vi "Test_WireLoops.vi"() -> ()   [LabVIEW 2025]
uses:
  8cebb4ce-4f0f-4319-9f7e-82e401bee674.vi
  Scripting Server.lvlib
panel:
  out "result":string
  in  "y":dbl
  out "error out":errorcluster
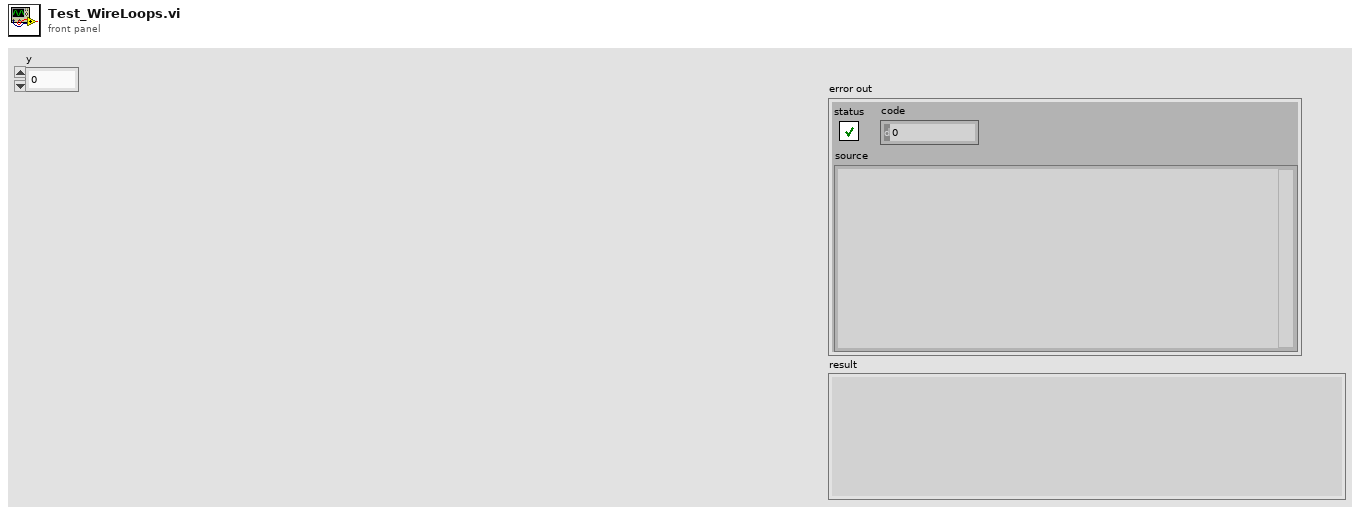
[diagram p1: front panel]
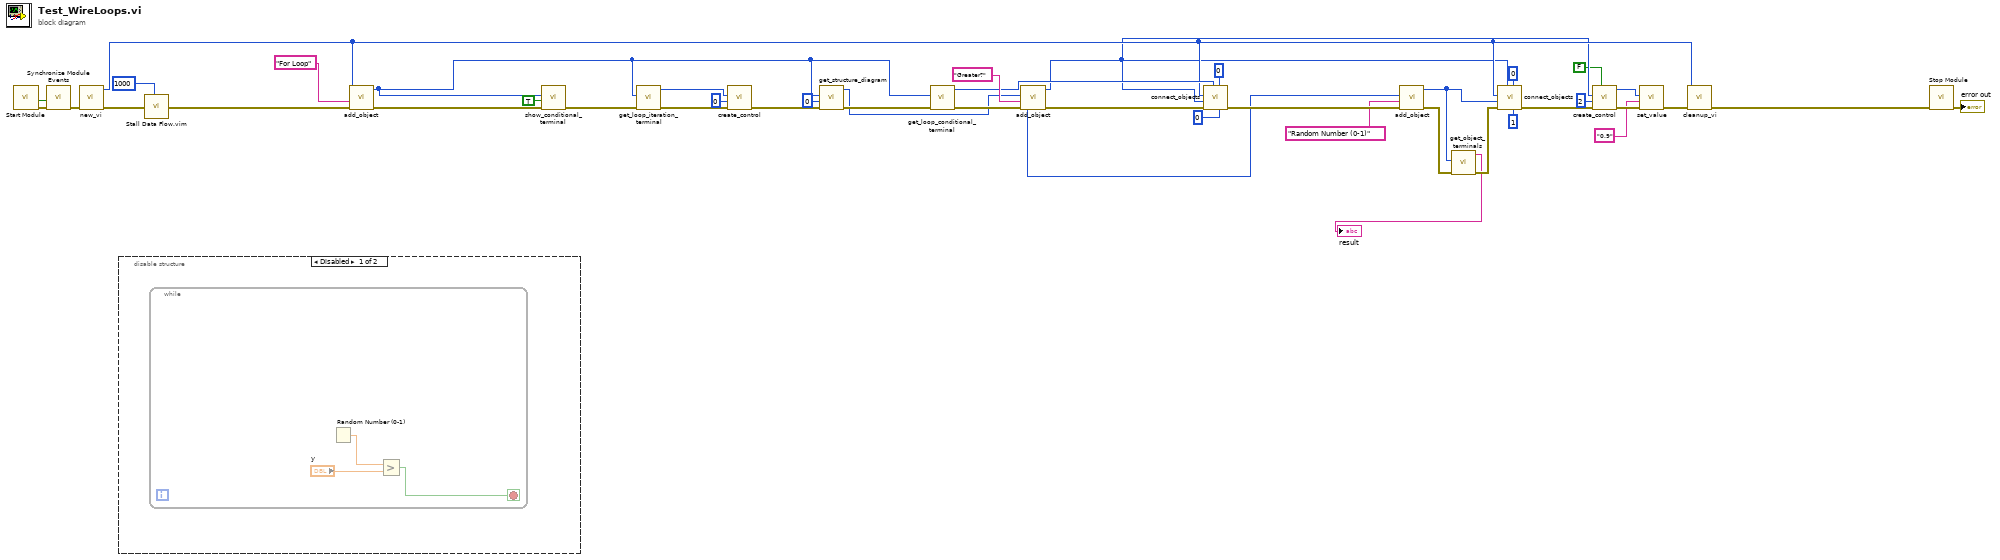
[diagram p0: block diagram]
diagram:
  n1 = call "Start Module.vi"() -> ("error out"=w42:errorcluster, "Wait for Event Sync?"=w43:bool)  [unwired: 7 in, 3 out]
  n2 = call "Synchronize Module Events.vi"("error in"=w42, "Wait for Event Sync?"=w43) -> ("error out"=w41:errorcluster)  [unwired: 9 in]
  n3 = call "new_vi.vi"("error in"=w41) -> ("error out"=w40:errorcluster, "vi_id"=w20:i32)  [unwired: 7 in, 2 out]
  n4 = disable-structure shown="Disabled" {
    frame Disabled {
      n5 = while {
        stop <- w44 stop-if-true
        n6 = Random Number (0-1)() -> (number: 0 to 1=w46:dbl)
        n7 = Greater?(x=w46, y="y") -> (0:w44:bool)
      }
    }
    frame Enabled {
    }
  }
  n8 = call "Stall Data Flow.vim"("value in"=w40, "milliseconds to wait"=u32 1000) -> ("value out"=w39:errorcluster)  [unwired: 1 out]
  n9 = call "add_object.vi"("error in"=w39, "object_name"="For Loop", "diagram_id"=w20) -> ("error out"=w35:errorcluster, "object_id"=w4:i32)  [unwired: 5 in, 2 out]
  n10 = call "show_conditional_terminal.vi"("error in"=w35, "show"=TRUE, "loop_id"=w4) -> ("error out"=w7:errorcluster)  [unwired: 7 in, 1 out]
  n11 = call "get_loop_iteration_terminal.vi"("error in"=w7, "loop_id"=w4) -> ("error out"=w5:errorcluster, "iteration_terminal_id"=w2:i32)  [unwired: 7 in, 1 out]
  n12 = call "create_control.vi"("error in"=w5, "terminal_index"=0, "object_id"=w2) -> ("error out"=w3:errorcluster)  [unwired: 6 in, 2 out]
  n13 = call "get_structure_diagram.vi"("error in"=w3, "index"=0, "structure_id"=w4) -> ("error out"=w29:errorcluster, "diagram_id"=w23:i32)  [unwired: 6 in, 1 out]
  n14 = call "get_loop_conditional_terminal.vi"("error in"=w29, "loop_id"=w4) -> ("error out"=w33:errorcluster, "conditional_terminal_id"=w27:i32)  [unwired: 7 in, 1 out]
  n15 = call "add_object.vi"("error in"=w33, "object_name"="Greater?", "diagram_id"=w23) -> ("error out"=w31:errorcluster, "object_id"=w16:i32)  [unwired: 5 in, 2 out]
  n16 = call "connect_objects.vi"("to_object_terminal_index"=0, "from_object_terminal_index"=0, "to_object_reference"=w27, "error in"=w31, "from_object_reference"=w16, "vi_reference"=w20) -> ("error out"=w32:errorcluster)  [unwired: 3 in, 2 out]
  n17 = call "add_object.vi"("error in"=w32, "object_name"="Random Number (0-1)", "diagram_id"=w23) -> ("error out"=w24:errorcluster, "object_id"=w9:i32)  [unwired: 5 in, 2 out]
  n18 = call "get_object_terminals.vi"("error in"=w24, "object_id"=w9) -> ("error out"=w10:errorcluster, "result"=→"result":string)  [unwired: 7 in, 1 out]
  n19 = call "connect_objects.vi"("to_object_terminal_index"=1, "from_object_terminal_index"=0, "to_object_reference"=w16, "error in"=w10, "from_object_reference"=w9, "vi_reference"=w20) -> ("error out"=w21:errorcluster)  [unwired: 3 in, 2 out]
  n20 = call "create_control.vi"("constant"=FALSE, "error in"=w21, "terminal_index"=2, "object_id"=w16) -> ("error out"=w17:errorcluster, "created_object_id"=w12:i32)  [unwired: 5 in, 1 out]
  n21 = call "set_value.vi"("error in"=w17, "value"="0.9", "object_id"=w12) -> ("error out"=w13:errorcluster)  [unwired: 7 in, 1 out]
  n22 = call "cleanup_vi.vi"("error in"=w13, "vi_reference"=w20) -> ("error out"=w36:errorcluster)  [unwired: 7 in, 2 out]
  n23 = call "Stop Module.vi"("error in"=w36) -> ("error out"=→"error out":errorcluster)  [unwired: 10 in]
